vi "ScpGetMeasMode.vi"(8 "error in (no error)":errorcluster, 11 "hDevice in":u32) -> (0 "error out":errorcluster, 1 "MeasureModeString":string, 2 "MeasureMode":u32, 3 "hDevice out":u32)   [LabVIEW 2018, in "LibTiePie.lvlib"]
uses:
  LibTiePie.lvlib
  LabViewHS4/libtiepie.dll
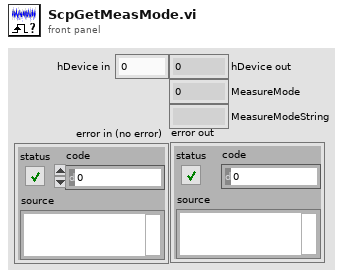
[diagram p1: front panel]
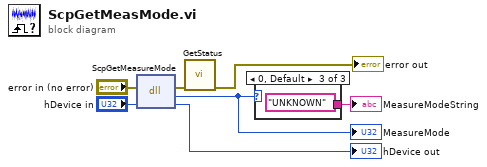
[diagram p0: block diagram]
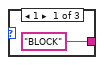
[diagram p2: hidden frame]
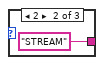
[diagram p3: hidden frame]
diagram:
  n1 = dll-call lib="C:/Users/cwaha/Documents/LabViewHS4/libtiepie.dll" fn="ScpGetMeasureMode"(error in="error in (no error)", "hDevice"="hDevice in") -> (error out=w7:errorcluster, "MeasureMode"=w6:u32, "hDevice"=→"hDevice out":u32)  [unwired: 2 in, 1 out]
  "MeasureMode" <- w6
  n2 = call "GetStatus.vi"("error in (no error)"=w7) -> ("error out"=→"error out":errorcluster)  [unwired: 10 in]
  n3 = case shown="0, Default" w6 {
    tunnel: ["BLOCK" "STREAM" "UNKNOWN"] -> w5
    frame 1 {
    }
    frame 2 {
    }
    frame 0, Default {
    }
  }
  "MeasureModeString" <- w5
